vi "Initialise.vi"(4 "Write Access":enum8{"Allowed", "Required", "None"}(ring), 6 "Read Access":enum8{"Allowed", "Required", "None"}(ring), 8 "error in (no error)":errorcluster, 10 "shared variable refnum":refnum<k21>, 11 "abs_SharedVar_Bool in":refnum<class "conc_SharedVar_U64.lvclass">) -> (0 "error out":errorcluster, 3 "abs_SharedVar_Bool out":refnum<class "conc_SharedVar_U64.lvclass">)   [LabVIEW 2021, in "conc_SharedVar_U64.lvclass"]
uses:
  conc_SharedVar_U64.lvclass
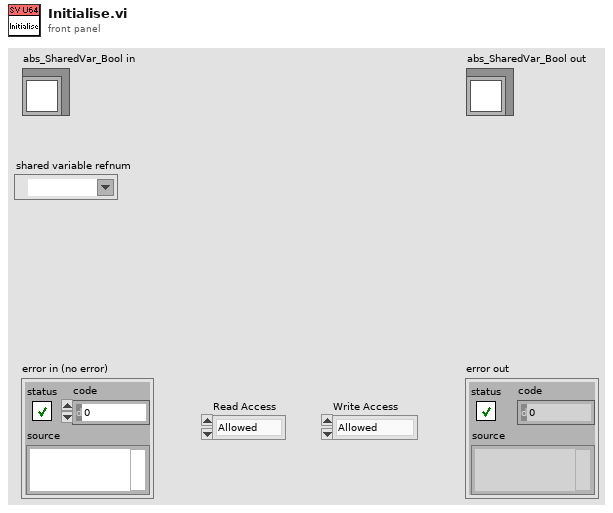
[diagram p1: front panel]
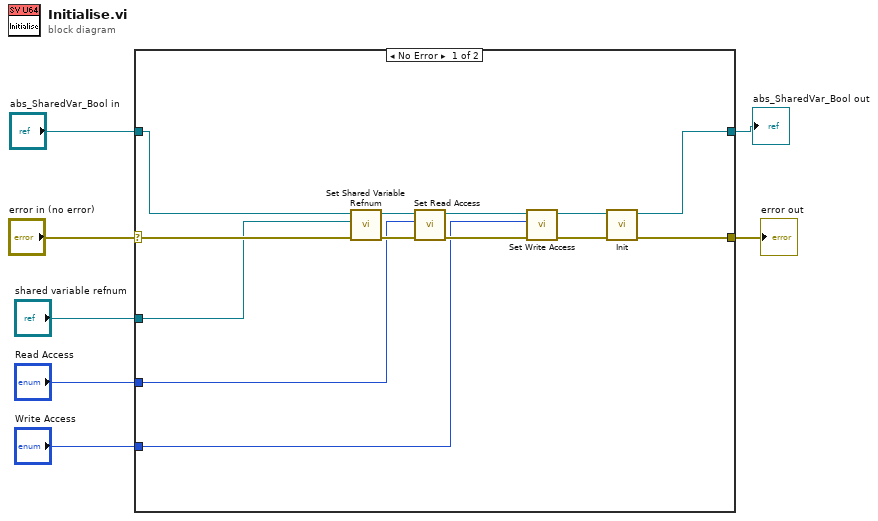
[diagram p0: block diagram]
diagram:
  n1 = case shown="No Error" "error in (no error)" {
    selector: "error in (no error)" -> [w18 w22]
    tunnel: [w20 w22] -> w6
    tunnel: [w19 w21] -> w4
    tunnel: "abs_SharedVar_Bool in" -> [w17 w21]
    tunnel: "Read Access" -> [w13 _]
    tunnel: "shared variable refnum" -> [w16 _]
    tunnel: "Write Access" -> [w10 _]
    frame No Error {
      n2 = call-dynamic "Set Shared Variable Refnum.vi"("error in (no error)"=w18, "shared variable refnum"=w16, "abs_SharedVar_Bool in"=w17) -> ("error out"=w15:errorcluster, "abs_SharedVar_Bool out"=w14:refnum<class "conc_SharedVar_U64.lvclass">)  [unwired: 7 in]
      n3 = call-dynamic "Set Read Access.vi"("error in (no error)"=w15, "Read Access"=w13, "abs_SharedVar_Bool in"=w14) -> ("error out"=w12:errorcluster, "abs_SharedVar_Bool out"=w11:refnum<class "conc_SharedVar_U64.lvclass">)  [unwired: 7 in]
      n4 = call-dynamic "Set Write Access.vi"("error in (no error)"=w12, "Write Access"=w10, "abs_SharedVar_Bool in"=w11) -> ("error out"=w9:errorcluster, "abs_SharedVar_Bool out"=w8:refnum<class "conc_SharedVar_U64.lvclass">)  [unwired: 7 in]
      n5 = call-dynamic "Init.vi"("error in (no error)"=w9, "Data in"=w8) -> ("error out"=w20:errorcluster, "Data out"=w19:refnum<class "conc_SharedVar_U64.lvclass">)  [unwired: 8 in]
    }
    frame Error {
    }
  }
  "error out" <- w6
  "abs_SharedVar_Bool out" <- w4
